vi "Client Main Async.vi"() -> ()   [LabVIEW 2012, in "Chat Client.lvclass"]
uses:
  Chat Client.lvclass
panel:
  out "Name":string
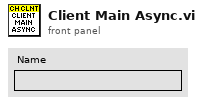
[diagram p1: front panel]
types:
  T1 = enum32{"Invalid", "Standard", "Closed", "Hidden", "Minimized", "Maximized"}
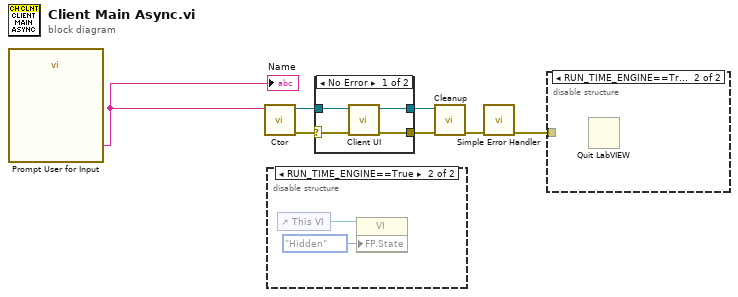
[diagram p0: block diagram]
diagram:
  n1 = call "Prompt User for Input"() -> ("Name"=w7:string)  [unwired: 17 in, 2 out]
  "Name" <- w7
  n2 = call "Ctor.vi"("Name"=w7) -> ("error out"=w6:errorcluster, "Chat Client out"=w5:refnum<class "Chat Client.lvclass">)  [unwired: 9 in]
  n3 = disable-structure shown="RUN_TIME_ENGINE==True" {
    frame condition #0 (active) {
    }
    frame condition #1 {
      n4 = control-ref of="This VI"() -> (w9:refnum<vi>)
      n5 = property class="VI"(reference=w9, "FP.State"=T1."Hidden" ("Front Panel Window:State")) -> ()  [unwired: 1 in, 2 out]
    }
  }
  n6 = case shown="No Error" w6 {
    selector: w6 -> [w12 w14]
    tunnel: w5 -> [w13 w15]
    tunnel: [w11 w15] -> w4
    tunnel: [w10 w14] -> w3
    frame No Error {
      n7 = call "Client UI.vi"("error in (no error)"=w12, "Chat Client in"=w13) -> ("error out"=w10:errorcluster, "Chat Client out"=w11:refnum<class "Chat Client.lvclass">)  [unwired: 8 in]
    }
    frame Error {
    }
  }
  n8 = call "Cleanup.vi"("error in (no error)"=w3, "Chat Client in"=w4) -> ("error out"=w2:errorcluster)  [unwired: 9 in]
  n9 = call <vilib>:"Simple Error Handler.vi"("error in (no error)"=w2) -> ("error out"=w1:errorcluster)  [unwired: 4 in, 4 out]
  n10 = disable-structure shown="RUN_TIME_ENGINE==True" {
    disable-tunnel: w1 -> [_ _]
    frame condition #0 (active) {
    }
    frame condition #1 {
      n11 = Quit LabVIEW() -> ()  [unwired: 1 in]
    }
  }
